vi "Main.vi"() -> ()   [LabVIEW 2024]
doc: "Main vi to run the Test Executive."
uses:
  <vilib>/Utility/miscctls.llb/LVRowAndColumnTypeDef.ctl
  <vilib>/addons/_JKI Toolkits/State Machine/_JKI_lib_State_Machine.llb/Select State(s)_err__jki_lib_state_machine.vi
  <vilib>/addons/_JKI Toolkits/State Machine/_JKI_lib_State_Machine.llb/Select State(s)_bool__jki_lib_state_machine.vi
  <vilib>/addons/_JKI Toolkits/State Machine/_JKI_lib_State_Machine.llb/Periodic Trigger__ogtk__JKI-SM__jki_lib_state_machine.vi
  <vilib>/Utility/file.llb/Read Delimited Spreadsheet (string).vi
  <userlib>/_OpenG.lib/file/file.llb/Strip Path Extension - String__ogtk.vi
  <userlib>/_OpenG.lib/lvzip/fileutil.llb/subVIs/FILE Rename (Path)__ogtk.vi
  <vilib>/Utility/file.llb/Write Delimited Spreadsheet (string).vi
  <vilib>/regexp/Match Regular Expression.xnode
  <userlib>/_OpenG.lib/appcontrol/appcontrol.llb/openg_application_control.lvlib
  <userlib>/_OpenG.lib/file/file.llb/openg_file.lvlib
  <userlib>/_OpenG.lib/string/string.llb/openg_string.lvlib
panel:
  in  "Abort Sequence":bool
  in  "Results":bool
  in  "TS Panel":bool
  in  "Tab Control":enum32{"TS", "R"}(tab)
  in  "SOF":bool caption="Checkbox"
  out "PassFail":string
  out "Sequence Name":string
  out "Status":string
  in  "Load Sequence":bool
  in  "Run Sequence":bool
  out "Sequence":string
  out "Operator":string
  out "Serial Number":string
  out "Results Table":string[][](table)
  in  "Exit":bool
  # "TEST EXECUTIVE V1"
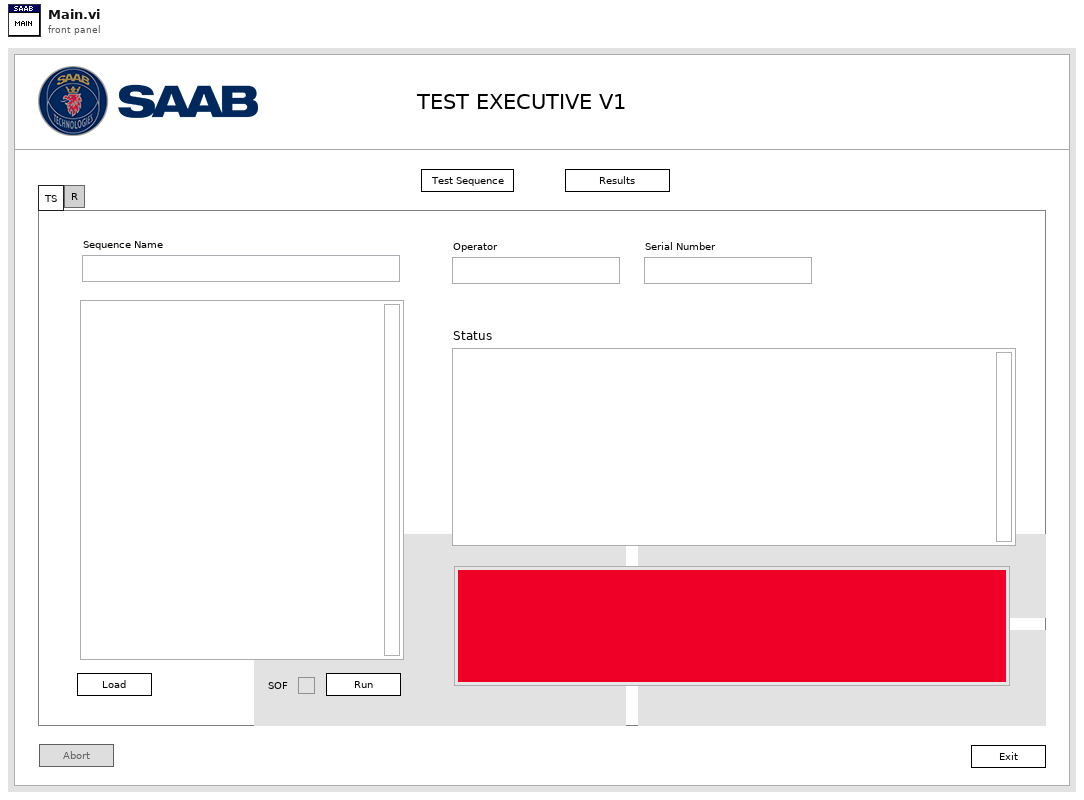
[diagram p1: front panel]
types:
  T1 = enum32{"Invalid", "Standard", "Closed", "Hidden", "Minimized", "Maximized"}
  T2 = enum32{"invalid app kind", "Development System", "Run Time System", "Student Edition", "Embedded LabVIEW", "Evaluation", "Custom"}
  T3 = cluster{"Core":cluster{"Current VI Reference":refnum<vi>, "Close Panel on Exit?":bool}, "Fail":bool, "Sequence Array":string[], "File Paths":cluster{"Seq File Path":path, "Limits File Path":path, "Results File Path":path, "Test File Path Array":path[]}, "Sequence Name":string, "Operator":string, "Serial Number":string, "Test Index":i32, "Test Time":dbl, "Start Seq TimeStamp ":cluster{"Start Seq Time":string, "Start Seq Date":string}, "End Seq Time":string, "Status":string, "SOF":bool, "Abort":bool, "Reference Array":refnum<vi>[]}
  T4 = cluster{"Start Seq Time":string, "Start Seq Date":string}
  T5 = cluster{"Seq File Path":path, "Limits File Path":path, "Results File Path":path, "Test File Path Array":path[]}
  T6 = cluster{"Current VI Reference":refnum<vi>, "Close Panel on Exit?":bool}
  T7 = enum8{"Enabled", "Disabled", "Disabled and Grayed Out"}
  T8 = typedef "LVRowAndColumnTypeDef.ctl" = cluster{"Row":i32, "Column":i32}
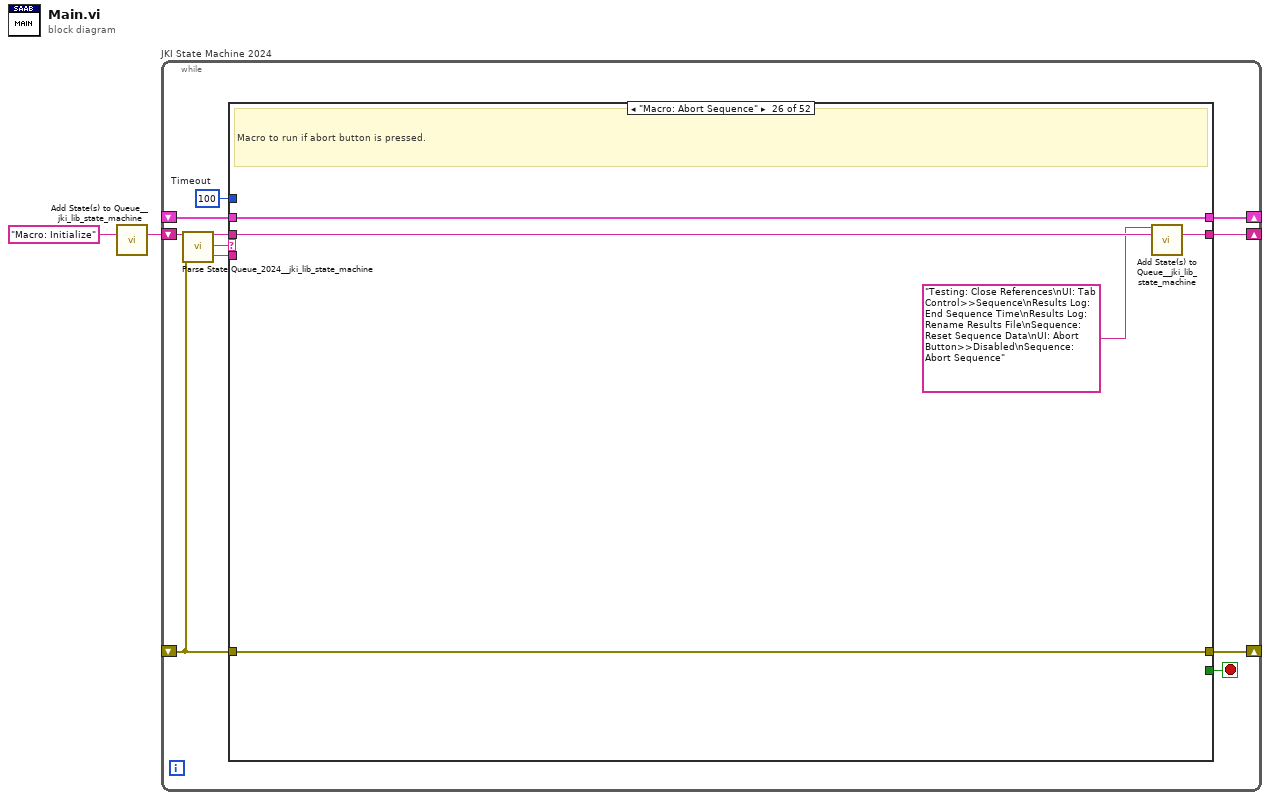
[diagram p0: block diagram]
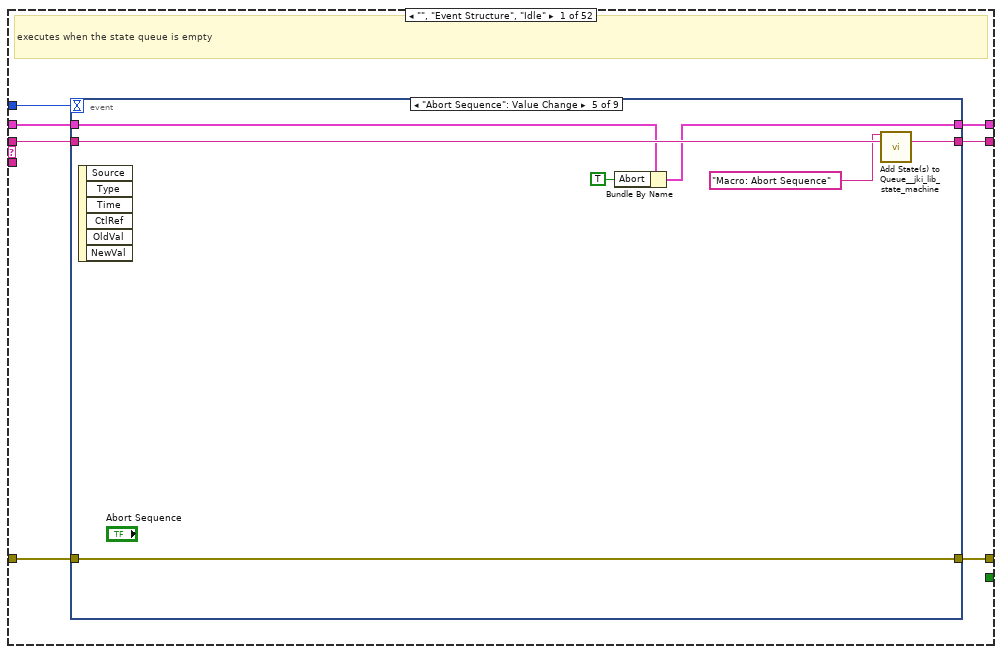
[diagram p2: hidden frame]
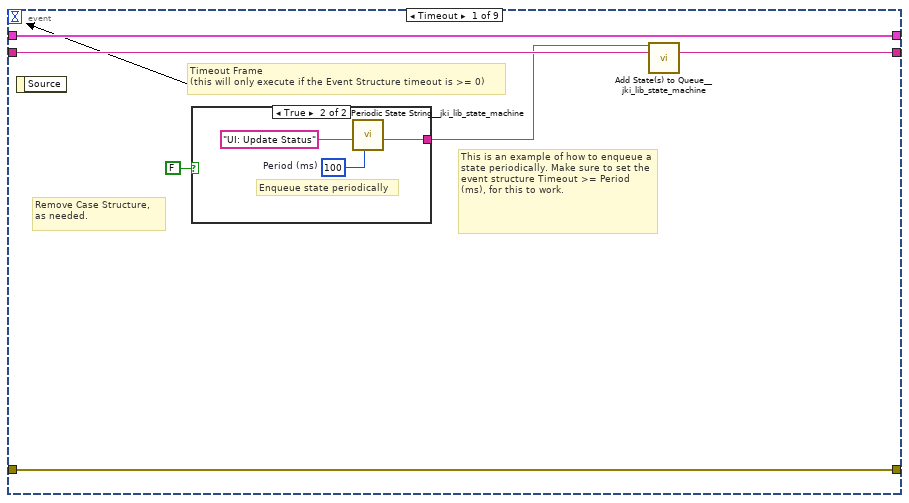
[diagram p3: hidden frame]
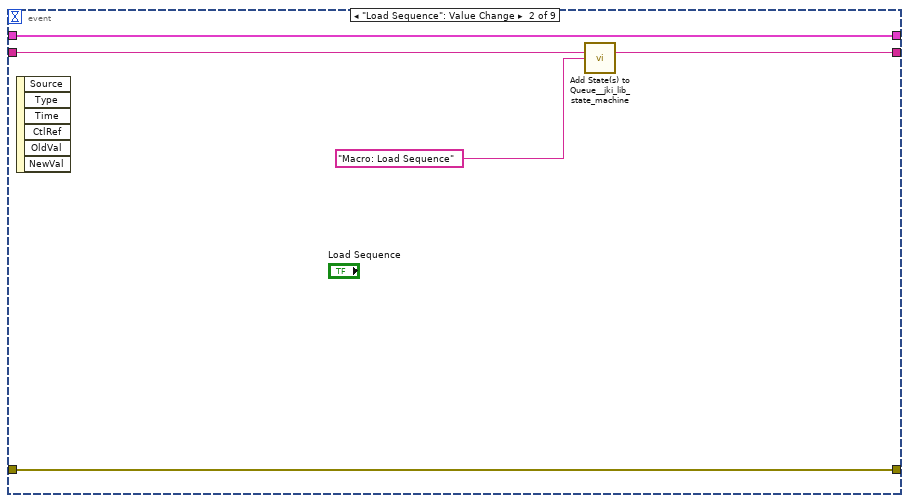
[diagram p5: hidden frame]
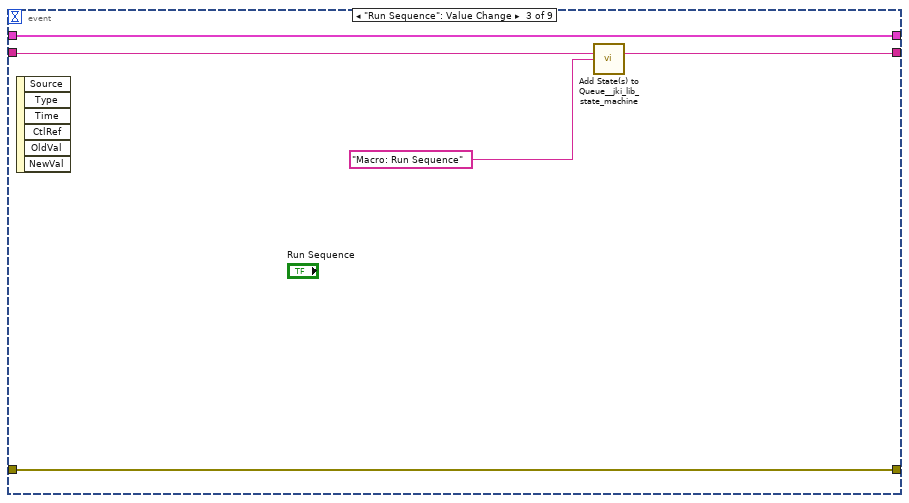
[diagram p6: hidden frame]
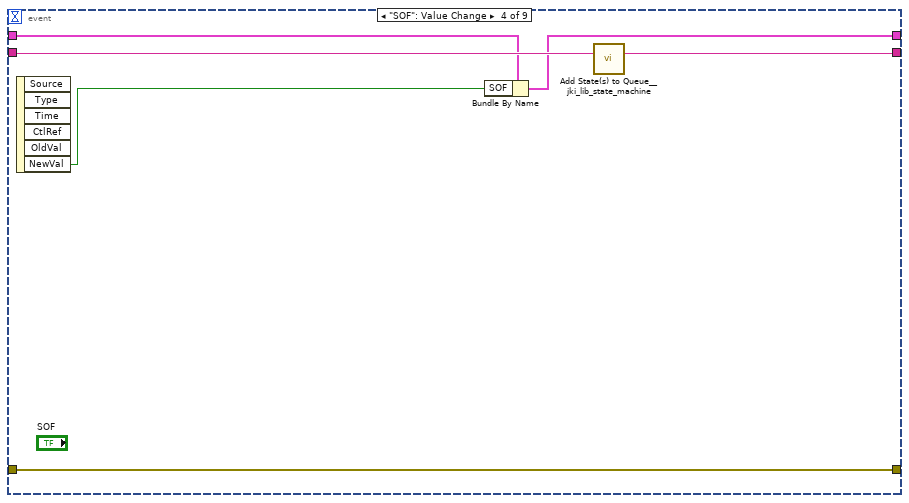
[diagram p7: hidden frame]
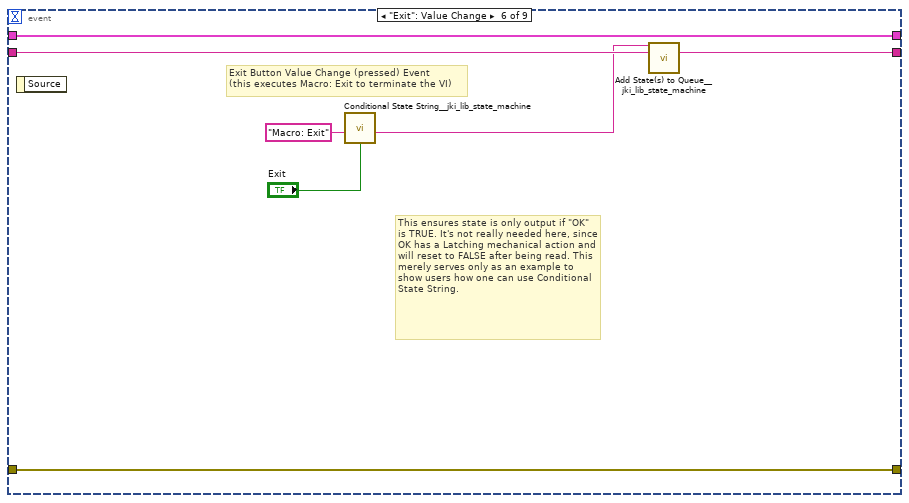
[diagram p8: hidden frame]
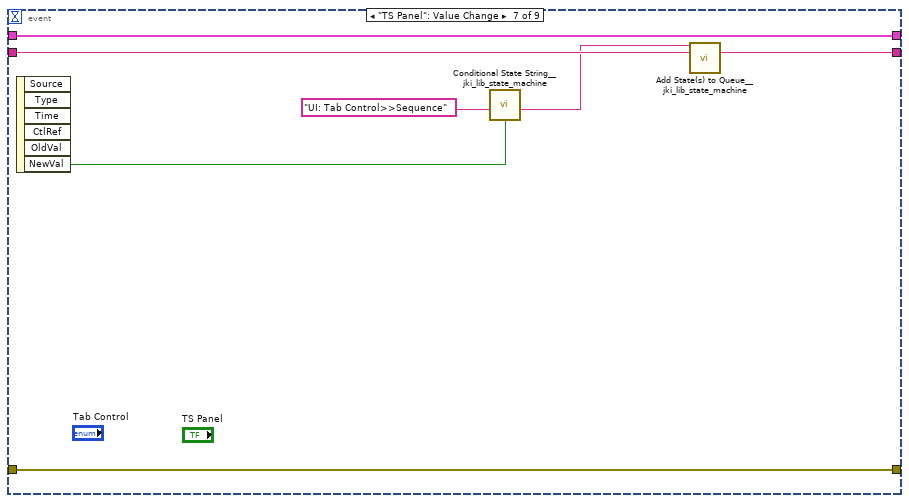
[diagram p9: hidden frame]
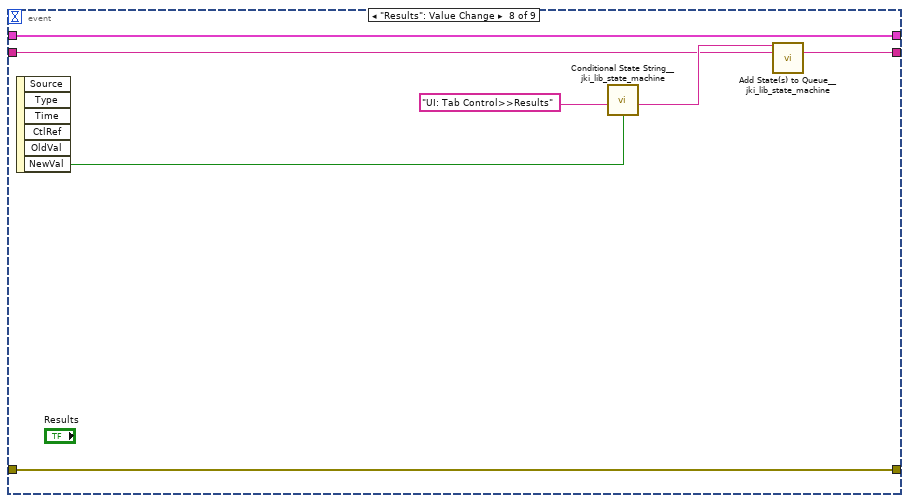
[diagram p10: hidden frame]
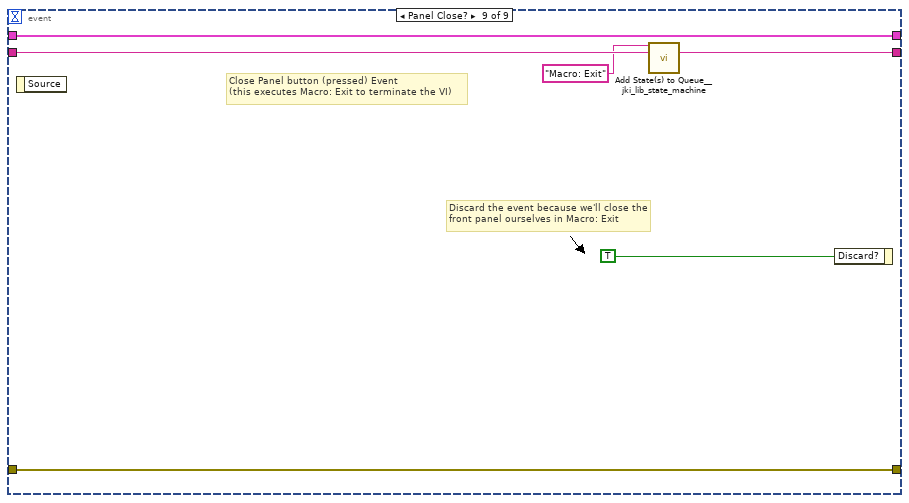
[diagram p11: hidden frame]
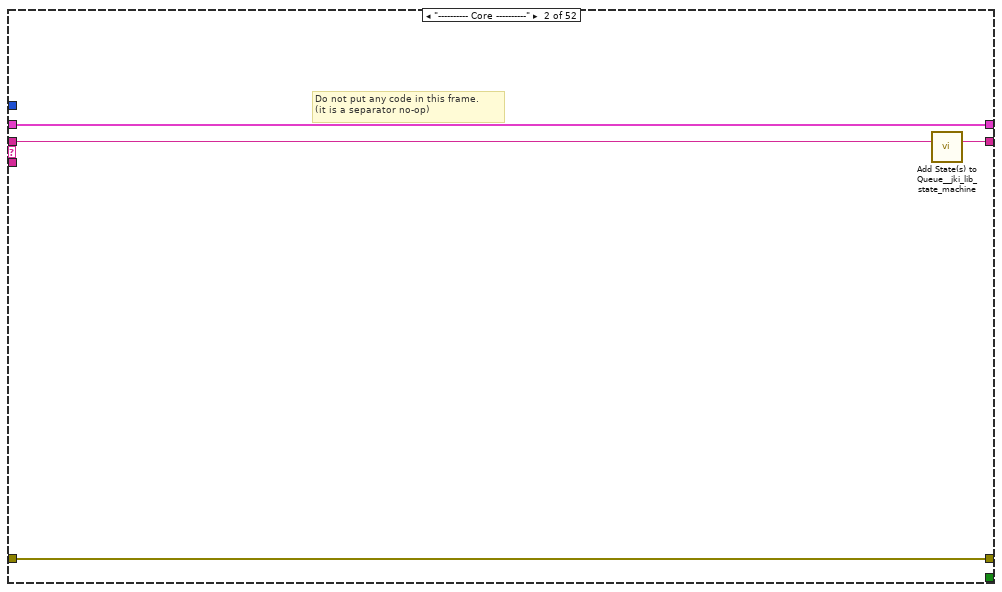
[diagram p12: hidden frame]
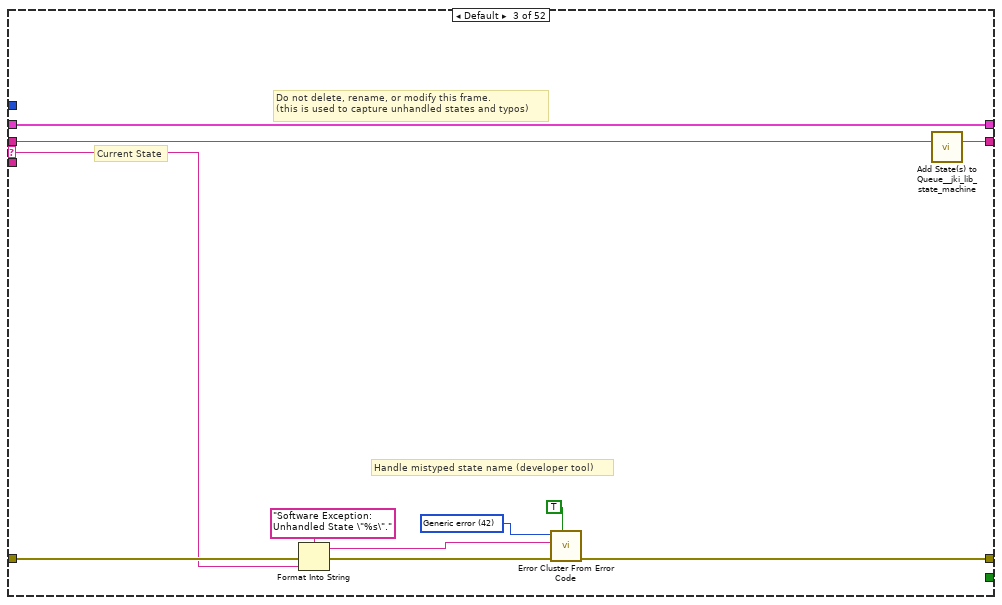
[diagram p13: hidden frame]
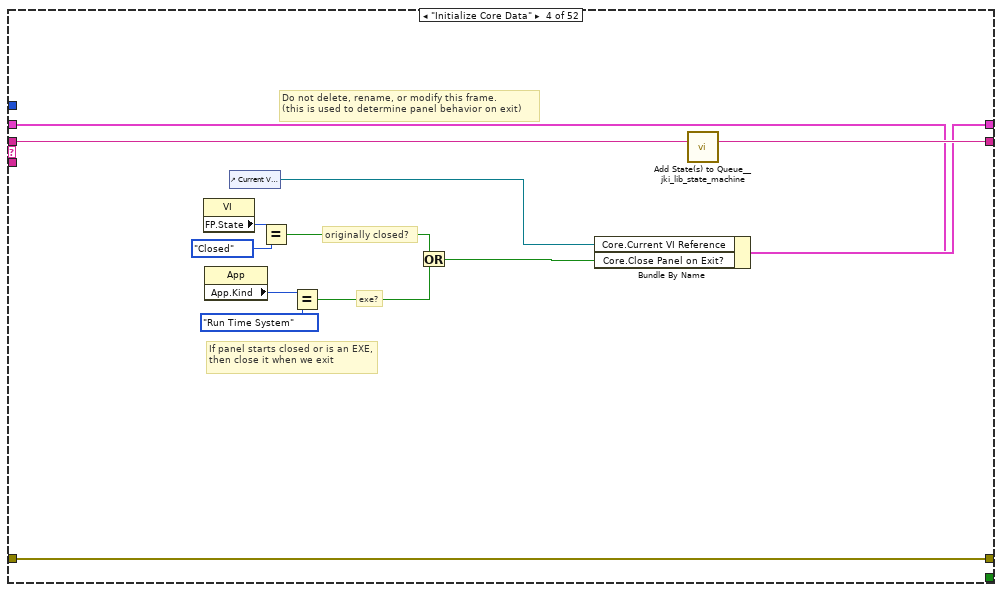
[diagram p14: hidden frame]
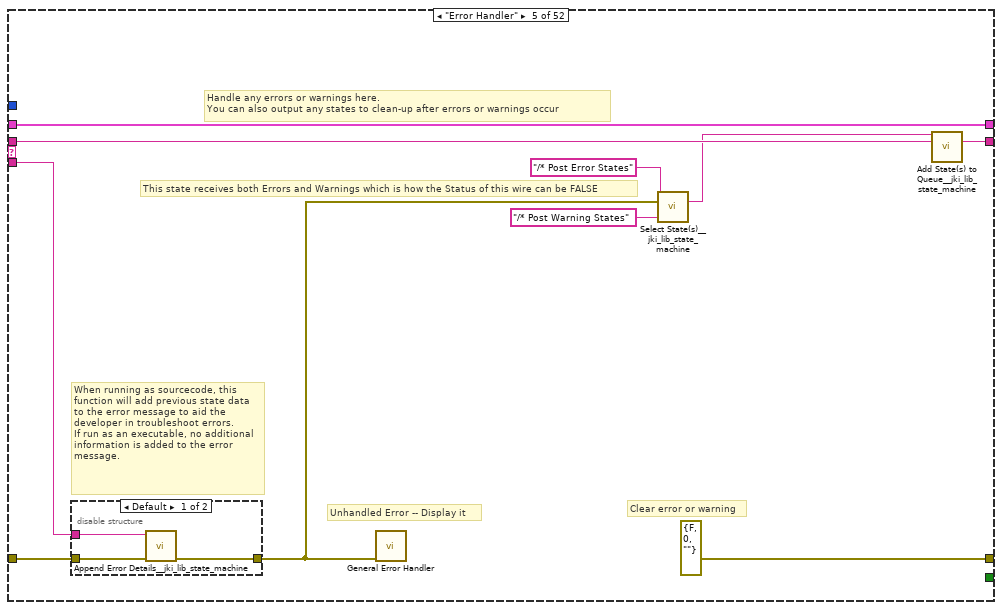
[diagram p15: hidden frame]
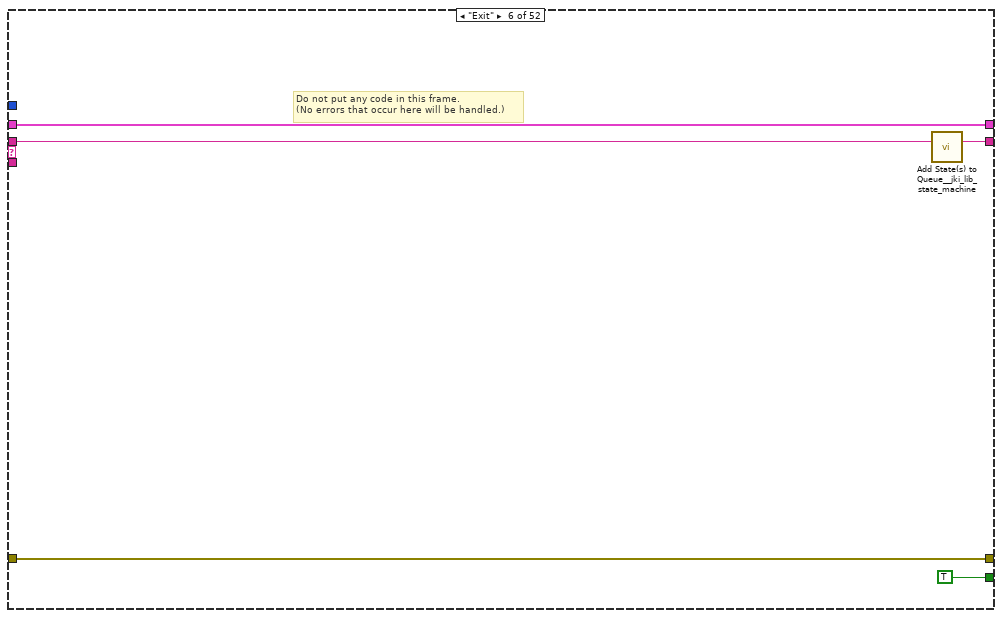
[diagram p17: hidden frame]
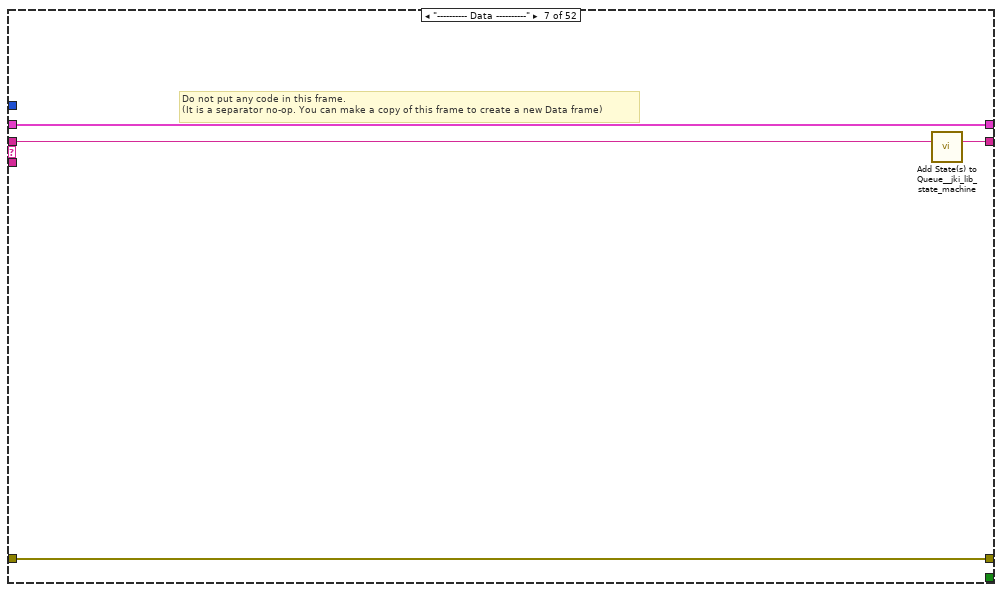
[diagram p18: hidden frame]
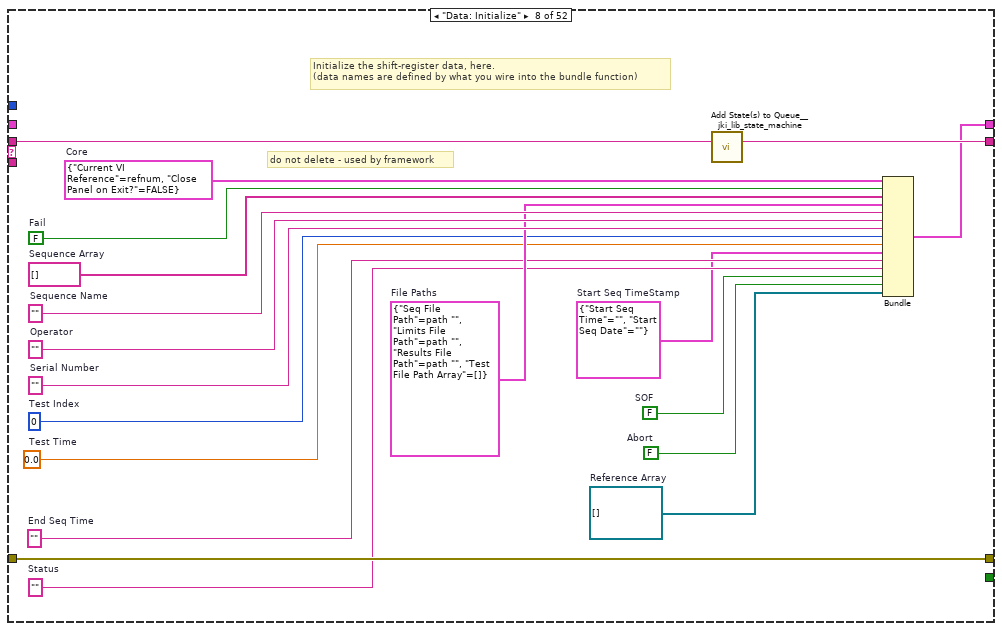
[diagram p19: hidden frame]
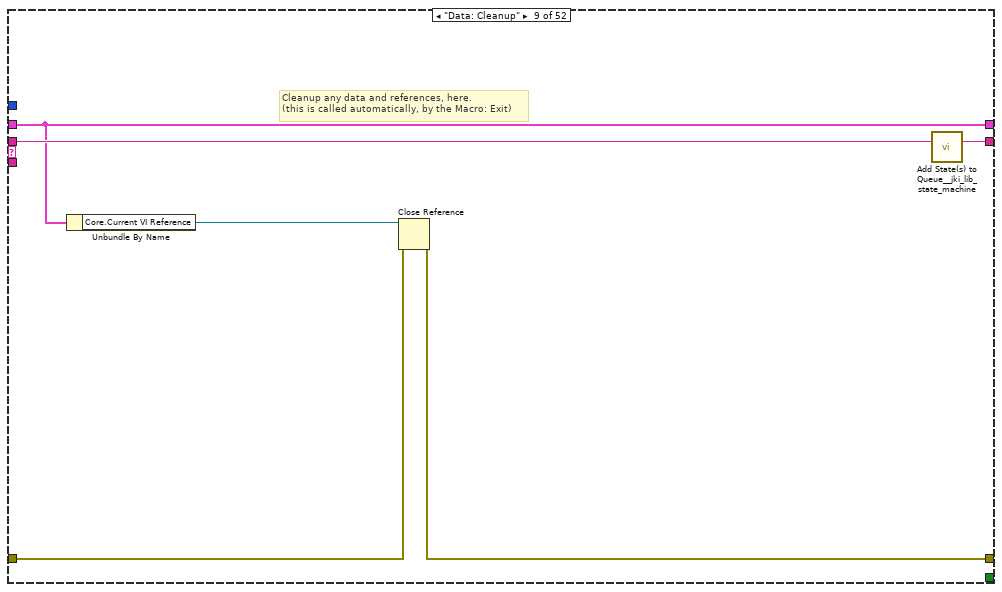
[diagram p20: hidden frame]
diagram:
  n1 = call <vilib>:"Add State(s) to Queue__jki_lib_state_machine.vi"("State(s) in (\"\")"="Macro: Initialize") -> ("States Out"=w2:string)  [unwired: 14 in]
  n2 = while "JKI State Machine 2024" {
    shift-right: [w6] -> _
    shift-left: _ -> [w5]
    shift-right: [w9] -> _
    shift-left: _ -> [w3]
    shift-right: [w8] -> _
    shift-left: w2 -> [w10]
    stop <- w7 stop-if-true
    w4 = 100  # Timeout
    n3 = call <vilib>:"Parse State Queue_2024__jki_lib_state_machine.vi"("State Queue"=w10, "Error In (no error)"=w3) -> ("Remaining States"=w12:string, "Current State"=w13:string, "Arguments"=w11:string)  [unwired: 11 in]
    n4 = case shown="\"Macro: Abort Sequence\"" w13 {
      selector: w13 -> [_ _ w84 _ _ _ _ _ _ _ _ _ _ _ _ _ _ _ _ _ _ _ _ _ _ _ _ _ _ _ _ _ _ _ _ _ _ _ _ _ _ _ _ _ _ _ _ _ _ _ _ _]
      tunnel: w12 -> [w20 w83 w88 w107 w117 w126 w130 w149 w155 w159 w169 w177 w195 w209 w220 w232 w241 w252 w258 w269 w338 w343 w348 w353 w358 w363 w368 w377 w381 w398 w413 w424 _ w431 w454 w462 w474 w492 w513 w522 w539 w580 w714 w731 w737 w755 w768 w783 w790 w799 w817 w825]
      tunnel: w11 -> [_ _ _ _ w112 _ _ _ _ _ _ w170 _ _ w215 _ _ w243 w253 w263 _ _ _ _ _ _ _ _ _ _ _ _ _ _ _ _ _ _ _ _ _ _ _ _ _ _ _ _ _ _ _ _]
      tunnel: w5 -> [w18 w80 w86 w100 w114 w124 w127 _ w150 w156 w167 w175 w192 w207 w218 w230 w239 w250 w256 w265 w335 w340 w345 w350 w354 w359 w365 w375 w378 w391 w408 w422 w425 w437 w452 w460 w471 w487 w511 w518 w528 w578 w710 w728 w744 w752 w765 w776 w786 w793 w807 w823]
      tunnel: [w17 w81 w90 w104 errorcluster {"status"=FALSE, "code"=0, "source"=""} ("error out") w123 w128 w144 w151 w157 w164 w174 w182 w205 w217 w223 w235 w249 w254 w266 w336 w341 w346 w351 w356 w361 w366 w372 w379 w385 w411 w420 w426 w433 w450 w455 w472 w489 w499 w520 w531 w562 w712 w722 w738 w753 w766 w781 w788 w797 w813 w820] -> w9
      tunnel: w3 -> [w14 w81 w89 w104 w113 w123 w128 w144 w152 w157 w162 w172 w193 w206 w216 w229 w238 w248 w255 w267 w336 w341 w346 w351 w356 w361 w366 w372 w379 w392 w411 w420 w429 w433 w450 w458 w472 w489 w510 w520 w534 w571 w712 w727 w742 w753 w766 w781 w788 w797 w812 w819]
      tunnel: [w19 w82 w87 w106 w116 w125 w129 w148 w154 w158 w168 w176 w194 w208 w219 w231 w240 w251 w257 w268 w337 w342 w347 w352 w357 w362 w367 w376 w380 w397 w412 w423 w430 w438 w453 w461 w473 w491 w512 w521 w538 w579 w713 w730 w745 w754 w767 w782 w789 w798 w816 w824] -> w8
      tunnel: [_ _ _ _ _ TRUE _ _ _ _ _ _ _ _ _ _ _ _ _ _ _ _ _ _ _ _ _ _ _ _ _ _ _ _ _ _ _ _ _ _ _ _ _ _ _ _ _ _ _ _ _ _] -> w7
      tunnel: [w16 w80 w86 w105 w114 w124 w127 w147 w150 w156 w167 w175 w192 w207 w218 w230 w239 w250 w256 w265 w335 w340 w345 w350 w354 w359 w365 w375 w378 w390 w408 w421 w425 w436 w451 w459 w471 w490 w511 w517 w527 w578 w709 w729 w743 w752 w765 w775 w785 w792 w806 w822] -> w6
      tunnel: w4 -> [w15 _ _ _ _ _ _ _ _ _ _ _ _ _ _ _ _ _ _ _ _ _ _ _ _ _ _ _ _ _ _ _ _ _ _ _ _ _ _ _ _ _ _ _ _ _ _ _ _ _ _ _]
      frame "", "Event Structure", "Idle" {
        # "executes when the state queue is empty"
        n5 = event shown="[4] \"Abort Sequence\": Value Change" {
          selector: _ -> [_ _ _ _ _ _ _ _ _]
          dyn-events: _ -> [_ _ _ _ _ _ _ _ _]
          timeout: w15 -> [_ _ _ _ _ _ _ _ _]
          tunnel: w20 -> [w26 w30 w37 w44 w50 w59 w64 w69 w79]
          tunnel: [w25 w33 w38 w45 w51 w58 w65 w71 w78] -> w19
          tunnel: w18 -> [w23 w31 w36 w41 w48 w56 w66 w73 w76]
          tunnel: [w24 w34 w35 w43 w52 w57 w60 w67 w77] -> w17
          tunnel: w14 -> [w24 w34 w35 w43 w52 w57 w60 w67 w77]
          tunnel: [w23 w31 w36 w42 w47 w56 w66 w73 w76] -> w16
          event Timeout {
            # "Remove Case Structure, as needed."
            # "This is an example of how to enqueue a state periodically. Make sure to set the event structure Timeout >= Period (ms), for this to work."
            # "Timeout Frame\n(this will only execute if the Event Structure timeout is >= 0)"
            n6 = event-data() -> ()  [unwired: 1 in, 1 out]
            n7 = case shown="True" FALSE {
              tunnel: [_ w29] -> w22
              frame False {
              }
              frame True {
                w27 = u32 100  # Period (ms)
                # "Enqueue state periodically"
                n8 = call <vilib>:"Periodic State String__jki_lib_state_machine.vi"("Period (ms)"=w27, "State"="UI: Update Status") -> ("State Out"=w29:string)  [unwired: 9 in]
              }
            }
            n9 = call <vilib>:"Add State(s) to Queue__jki_lib_state_machine.vi"("State(s) in Front (\"\")"=w22, "State(s) in (\"\")"=w26) -> ("States Out"=w25:string)  [unwired: 13 in]
          }
          event "Load Sequence": Value Change {
            n10 = event-data() -> ()  [unwired: 1 in, 6 out]
            n11 = call <vilib>:"Add State(s) to Queue__jki_lib_state_machine.vi"("State(s) in (\"\")"=w30, "State(s) at Back (\"\")"="Macro: Load Sequence" ("State(s) at Back (\"\")")) -> ("States Out"=w33:string)  [unwired: 13 in]
          }
          event "Run Sequence": Value Change {
            n12 = event-data() -> ()  [unwired: 1 in, 6 out]
            n13 = call <vilib>:"Add State(s) to Queue__jki_lib_state_machine.vi"("State(s) in (\"\")"=w37, "State(s) at Back (\"\")"="Macro: Run Sequence" ("State(s) at Back (\"\")")) -> ("States Out"=w38:string)  [unwired: 13 in]
          }
          event "SOF": Value Change {
            n14 = event-data() -> ("NewVal"=w40:bool)  [unwired: 1 in, 5 out]
            n15 = Bundle By Name(cluster=w41, "SOF"=w40) -> (w42:T3)
            n16 = call <vilib>:"Add State(s) to Queue__jki_lib_state_machine.vi"("State(s) in (\"\")"=w44) -> ("States Out"=w45:string)  [unwired: 14 in]
          }
          event "Abort Sequence": Value Change {
            n17 = event-data() -> ()  [unwired: 1 in, 6 out]
            n18 = Bundle By Name(cluster=w48, "Abort"=TRUE) -> (w47:T3)
            n19 = call <vilib>:"Add State(s) to Queue__jki_lib_state_machine.vi"("State(s) in Front (\"\")"="Macro: Abort Sequence", "State(s) in (\"\")"=w50) -> ("States Out"=w51:string)  [unwired: 13 in]
          }
          event "Exit": Value Change {
            # "This ensures state is only output if \"OK\" is TRUE. It's not really needed here, since OK has a Latching mechanical action and will reset to FALSE after being read. This merely serves only as an example to show users how one can use Conditional State String."
            # "Exit Button Value Change (pressed) Event\n(this executes Macro: Exit to terminate the VI)"
            n20 = event-data() -> ()  [unwired: 1 in, 1 out]
            n21 = call <vilib>:"Conditional State String__jki_lib_state_machine.vi"("Do State(s)?"="Exit", "State"="Macro: Exit") -> ("State Out"=w53:string)  [unwired: 7 in]
            n22 = call <vilib>:"Add State(s) to Queue__jki_lib_state_machine.vi"("State(s) in Front (\"\")"=w53, "State(s) in (\"\")"=w59) -> ("States Out"=w58:string)  [unwired: 13 in]
          }
          event "TS Panel": Value Change {
            n23 = event-data() -> ("NewVal"=w62:bool)  [unwired: 1 in, 5 out]
            n24 = call <vilib>:"Conditional State String__jki_lib_state_machine.vi"("Do State(s)?"=w62, "State"="UI: Tab Control>>Sequence") -> ("State Out"=w63:string)  [unwired: 7 in]
            n25 = call <vilib>:"Add State(s) to Queue__jki_lib_state_machine.vi"("State(s) in Front (\"\")"=w63, "State(s) in (\"\")"=w64) -> ("States Out"=w65:string)  [unwired: 13 in]
          }
          event "Results": Value Change {
            n26 = event-data() -> ("NewVal"=w68:bool)  [unwired: 1 in, 5 out]
            n27 = call <vilib>:"Conditional State String__jki_lib_state_machine.vi"("Do State(s)?"=w68, "State"="UI: Tab Control>>Results") -> ("State Out"=w70:string)  [unwired: 7 in]
            n28 = call <vilib>:"Add State(s) to Queue__jki_lib_state_machine.vi"("State(s) in Front (\"\")"=w70, "State(s) in (\"\")"=w69) -> ("States Out"=w71:string)  [unwired: 13 in]
          }
          event Panel Close? {
            # "Discard the event because we'll close the front panel ourselves in Macro: Exit"
            # "Close Panel button (pressed) Event\n(this executes Macro: Exit to terminate the VI)"
            n29 = event-data() -> ()  [unwired: 1 in, 1 out]
            n30 = call <vilib>:"Add State(s) to Queue__jki_lib_state_machine.vi"("State(s) in Front (\"\")"="Macro: Exit", "State(s) in (\"\")"=w79) -> ("States Out"=w78:string)  [unwired: 13 in]
            n31 = event-data("Discard?"=TRUE) -> ()  [unwired: 1 in, 1 out]
          }
        }
      }
      frame "---------- Core ----------" {
        # "Do not put any code in this frame.\n(it is a separator no-op)"
        n32 = call <vilib>:"Add State(s) to Queue__jki_lib_state_machine.vi"("State(s) in (\"\")"=w83) -> ("States Out"=w82:string)  [unwired: 14 in]
      }
      frame Default {
        w93 = 42 items=["No error", "Argument error", "Memory is full", "Out of zone", "End of file", "File already open", "Generic file I/O error", "File not found", "File permission error", "Disk is full", "Duplicate path", "Too many files open", "System feature not enabled", "Resource file not found", "Cannot add resource", "Resource not found", "Image not found", "Image memory error", "Pen does not exist", "Config type invalid", "Config token not found", "Config parse error", "Config memory error", "Bad external code format", "Bad external code offset", "External code not present", "Null window", "Destroy window error", "Null menu", "Print aborted", "Bad print record", "Print driver error", "Windows error during printing", "Memory error during printing", "Print dialog error", "Generic print error", "Invalid device refnum", "Device not found", "Device parameter error", "Device unit error", "Cannot open device", "Device call aborted", "Generic error", "Cancelled by user", "Object ID too low", "Object ID too high", "Object not in heap", "Unknown heap", "Unknown object (invalid DefProc)", "Unknown object (DefProc not in table)", "Message out of range", "Invalid (null) method", "Unknown message", "Manager call not supported", "Bad address", "Network operation in progress", "Network operation timed out", "Connection is busy", "Network attribute not supported", "Network error", "Address in use", "System out of memory", "Connection aborted", "Connection refused", "Not connected", "Already connected", "Connection closed", "Initialization error (interapplication manager)", "Bad occurrence", "Wait on unbound occurrence handler", "Occurrence queue overflow", "Datalog type conflict", "Unused", "Unrecognized type (interapplication manager)", "Memory corrupt", "Failed to make temporary DLL", "Old CIN version", "Drag socket not found", "Failed to load drop-object", "Failed to register OLE object", "Failed to release OLE object", "Format specifier type mismatch", "Unknown format specifier", "Too few format specifiers", "Too many format specifiers", "Scan failed", "Newer CIN version", "Error converting to variant", "Runtime menu error", "Password tampered", "Variant attribute not found", "Incompatible variant data type", "Event data is not available", "Event Store is not present", "Occurrence is not found", "Event Queue is not created", "Event info is not available", "Refnum passed is NULL", "Error retrieving Class GUID", "Error retrieving CoClass GUID", "Error retrieving TypeLib GUID.", "Bad built application magic bytes.", "Specific driver is different from the specific driver associated with the Logical Name.", "There is no session opened to the class driver.", "Max Error", "MAX - Error with config objects", "MAX - Error loading configuration", "MAX - Group not supported"]
        # "Current State"
        # "Do not delete, rename, or modify this frame.\n(this is used to capture unhandled states and typos)"
        # "Handle mistyped state name (developer tool)"
        n33 = Format Into String(format string="Software Exception: Unhandled State \"%s\"." ("message"), error in=w89, w84) -> (resulting string=w92:string, error out=w91:errorcluster)  [unwired: 1 in]
        n34 = call <vilib>:"Error Cluster From Error Code.vi"("show call chain? (False)"=TRUE, "error in (no error)"=w91, "error message (\"\")"=w92, "error code (0)"=w93) -> ("error out"=w90:errorcluster)  [unwired: 5 in]
        n35 = call <vilib>:"Add State(s) to Queue__jki_lib_state_machine.vi"("State(s) in (\"\")"=w88) -> ("States Out"=w87:string)  [unwired: 14 in]
      }
      frame "Initialize Core Data" {
        # "Do not delete, rename, or modify this frame.\n(this is used to determine panel behavior on exit)"
        # "originally closed?"
        # "exe?"
        # "If panel starts closed or is an EXE, then close it when we exit"
        n36 = property class="VI"() -> ("FP.State"=w97:T1)  [unwired: 2 in, 2 out]
        n37 = property class="App"() -> ("App.Kind"=w103:T2)  [unwired: 2 in, 2 out]
        n38 = control-ref of="Current VI Reference"() -> (w98:refnum<vi>)
        n39 = Equal?(x=w97, y=T1."Closed" ("Front Panel Window:State")) -> (x = y?=w95:bool)
        n40 = Equal?(x=w103, y=T2."Run Time System" ("Application:Kind")) -> (x = y?=w101:bool)
        n41 = Or(x=w95, y=w101) -> (x .or. y?=w99:bool)
        n42 = Bundle By Name(cluster=w100, "Core.Current VI Reference"=w98, "Core.Close Panel on Exit?"=w99) -> (w105:T3)
        n43 = call <vilib>:"Add State(s) to Queue__jki_lib_state_machine.vi"("State(s) in (\"\")"=w107) -> ("States Out"=w106:string)  [unwired: 14 in]
      }
      frame "Error Handler" {
        # "When running as sourcecode, this function will add previous state data to the error message to aid the developer in troubleshoot errors.\nIf run as an executable, no additional information is added to the error message."
        # "This state receives both Errors and Warnings which is how the Status of this wire can be FALSE"
        # "Unhandled Error -- Display it"
        # "Handle any errors or warnings here.\nYou can also output any states to clean-up after errors or warnings occur"
        # "Clear error or warning"
        n44 = disable-structure shown="Default" {
          disable-tunnel: w113 -> [w120 w121]
          disable-tunnel: w112 -> [w119 _]
          disable-tunnel: [w118 w121] -> w111
          frame condition #0 (active) {
            n45 = call <vilib>:"Append Error Details__jki_lib_state_machine.vi"("error in (no error)"=w120, "Previous State and Argument(s)"=w119) -> ("error out"=w118:errorcluster)  [unwired: 9 in]
          }
          frame condition #1 {
          }
        }
        n46 = call <vilib>:"General Error Handler.vi"("error in (no error)"=w111) -> ()  [unwired: 10 in, 5 out]
        n47 = call-poly <vilib>:"Select State(s)__jki_lib_state_machine.vi"("State(s) if True (\"\")"="/* Post Error States", "Select"=w111, "State(s) if False (\"\")"="/* Post Warning States") -> ("States Out"=w109:string)  [unwired: 12 in]
        n48 = call <vilib>:"Add State(s) to Queue__jki_lib_state_machine.vi"("State(s) in Front (\"\")"=w109, "State(s) in (\"\")"=w117) -> ("States Out"=w116:string)  [unwired: 13 in]
      }
      frame "Exit" {
        # "Do not put any code in this frame.\n(No errors that occur here will be handled.)"
        n49 = call <vilib>:"Add State(s) to Queue__jki_lib_state_machine.vi"("State(s) in (\"\")"=w126) -> ("States Out"=w125:string)  [unwired: 14 in]
      }
      frame "---------- Data ----------" {
        # "Do not put any code in this frame.\n(It is a separator no-op. You can make a copy of this frame to create a new Data frame)"
        n50 = call <vilib>:"Add State(s) to Queue__jki_lib_state_machine.vi"("State(s) in (\"\")"=w130) -> ("States Out"=w129:string)  [unwired: 14 in]
      }
      frame "Data: Initialize" {
        w131 = refnum<vi>[] []  # Reference Array
        w132 = FALSE  # Abort
        w133 = FALSE  # SOF
        w134 = T4 {"Start Seq Time"="", "Start Seq Date"=""}  # Start Seq TimeStamp
        w135 = ""  # Status
        w136 = ""  # End Seq Time
        w137 = 0.0  # Test Time
        w138 = 0  # Test Index
        w139 = T5 {"Seq File Path"=path "", "Limits File Path"=path "", "Results File Path"=path "", "Test File Path Array"=[]}  # File Paths
        w140 = string[] []  # Sequence Array
        w141 = ""  # Serial Number
        w142 = ""  # Operator
        w143 = ""  # Sequence Name
        w145 = T6 {"Current VI Reference"=refnum, "Close Panel on Exit?"=FALSE}  # Core
        w146 = FALSE  # Fail
        # "do not delete - used by framework"
        # "Initialize the shift-register data, here.\n(data names are defined by what you wire into the bundle function)"
        n51 = call <vilib>:"Add State(s) to Queue__jki_lib_state_machine.vi"("State(s) in (\"\")"=w149) -> ("States Out"=w148:string)  [unwired: 14 in]
        n52 = Bundle("Core"=w145, "Fail"=w146, "Sequence Array"=w140, "File Paths"=w139, "Sequence Name"=w143, "Operator"=w142, "Serial Number"=w141, "Test Index"=w138, "Test Time"=w137, "Start Seq TimeStamp"=w134, "End Seq Time"=w136, "Status"=w135, "SOF"=w133, "Abort"=w132, "Reference Array"=w131) -> (w147:T3)  [unwired: 1 in]
      }
      frame "Data: Cleanup" {
        # "Cleanup any data and references, here.\n(this is called automatically, by the Macro: Exit)"
        n53 = Unbundle By Name(w150) -> ("Core.Current VI Reference"=w153:refnum<vi>)
        n54 = Close Reference(reference=w153, error in (no error)=w152) -> (error out=w151:errorcluster)
        n55 = call <vilib>:"Add State(s) to Queue__jki_lib_state_machine.vi"("State(s) in (\"\")"=w155) -> ("States Out"=w154:string)  [unwired: 14 in]
      }
      frame "---------- UI ----------" {
        # "Do not put any code in this frame.\n(It is a separator no-op. You can make a copy of this frame to create a new UI frame)"
        n56 = call <vilib>:"Add State(s) to Queue__jki_lib_state_machine.vi"("State(s) in (\"\")"=w159) -> ("States Out"=w158:string)  [unwired: 14 in]
      }
      frame "UI: Initialize" {
        w160 = FALSE  # SOF
        w163 = enum32{"TS", "R"}."TS"  # Tab Control
        # "Initialize the User Interface, here.\n(this is called automatically, by the Macro: Initialize)"
        n57 = property on="SOF" class="Bool (strict)"(error in=w162, "Value"=w160) -> (error out=w161:errorcluster)  [unwired: 1 in, 1 out]
        n58 = property on="Tab Control" class="TabCtl (strict)"(error in=w161, "Tabs Visible?"=FALSE, "Value"=w163) -> (error out=w165:errorcluster)  [unwired: 1 in, 1 out]
        n59 = call <userlib>:"Fit VI window to Largest Dec__ogtk.vi"("error in (no error)"=w165) -> ("error out"=w164:errorcluster)  [unwired: 5 in, 1 out]
        n60 = call <vilib>:"Add State(s) to Queue__jki_lib_state_machine.vi"("State(s) in (\"\")"=w169) -> ("States Out"=w168:string)  [unwired: 14 in]
      }
      frame "UI: Tab Control" {
        # "Selects the tab defined by the state argument"
        n61 = case shown="\"Sequence\", Default" w170 {
          tunnel: [w179 w181] -> w173
          tunnel: w172 -> [w178 w180]
          tunnel: [w178 w180] -> w171
          frame "Results" {
            w179 = enum32{"TS", "R"}."R"  # Tab Control
          }
          frame "Sequence", Default {
            w181 = enum32{"TS", "R"}."TS"  # Tab Control
          }
        }
        n62 = property on="Tab Control" class="TabCtl (strict)"(error in=w171, "Value"=w173) -> (error out=w174:errorcluster)  [unwired: 1 in, 1 out]
        n63 = call <vilib>:"Add State(s) to Queue__jki_lib_state_machine.vi"("State(s) in (\"\")"=w177) -> ("States Out"=w176:string)  [unwired: 14 in]
      }
      frame "UI: Update Status" {
        # "Update the status on the FP. Build the text for the status string and add any failures. Display a big passfail string box and colour appropriatly."
        n64 = Unbundle By Name(w192) -> ("Start Seq TimeStamp.Start Seq Date"=w190:string, "Start Seq TimeStamp.Start Seq Time"=w189:string, "End Seq Time"=w188:string, "File Paths.Results File Path"=w191:path)
        n65 = call "Search for Fail.vi"("Results File Path"=w191, "error in (no error)"=w193) -> ("String"=w186:string, "Pass Status"=w184:bool, "error out"=w185:errorcluster)  [unwired: 11 in]
        n66 = case shown="False" w184 {
          tunnel: w185 -> [w198 w202]
          tunnel: ["FAIL" "PASS"] -> w183
          tunnel: [w197 w201] -> w182
          frame False {
            n67 = property on="PassFail" class="Str"(error in=w198, "Text.BGColor"=u32 15663143) -> (error out=w197:errorcluster)  [unwired: 1 in, 1 out]
          }
          frame True {
            n68 = property on="PassFail" class="Str"(error in=w202, "Text.BGColor"=u32 51250) -> (error out=w201:errorcluster)  [unwired: 1 in, 1 out]
          }
        }
        "PassFail" <- w183
        n69 = call "Build Text2"("Fail"=w186, "Date"=w190, "Start"=w189, "Finish"=w188) -> ("Result"=→"Status":string)  [unwired: 10 in, 1 out]
        n70 = call <vilib>:"Add State(s) to Queue__jki_lib_state_machine.vi"("State(s) in (\"\")"=w195) -> ("States Out"=w194:string)  [unwired: 14 in]
      }
      frame "UI: Uninitialize" {
        # "Cleanup the User Interface, here.\n(this is called automatically, by the Macro: Exit)"
        n71 = property on="Tab Control" class="TabCtl (strict)"(error in=w206, "Tabs Visible?"=TRUE) -> (error out=w205:errorcluster)  [unwired: 1 in, 1 out]
        n72 = call <vilib>:"Add State(s) to Queue__jki_lib_state_machine.vi"("State(s) in (\"\")"=w209) -> ("States Out"=w208:string)  [unwired: 14 in]
      }
      frame "UI: Run Button" {
        w212 = T7."Disabled and Grayed Out"  # Disabled
        w213 = T7."Enabled"  # Disabled
        # "Enables or disabled the Run button based on state arguments."
        n73 = Equal?(x=w215, y="Disabled") -> (x = y?=w214:bool)
        n74 = Select(t=w212, s=w214, f=w213) -> (s? t:f=w210:T7)
        n75 = property on="Run Sequence" class="Bool"(error in=w216, "DisabledEnum"=w210) -> (error out=w217:errorcluster)  [unwired: 1 in, 1 out]
        n76 = call <vilib>:"Add State(s) to Queue__jki_lib_state_machine.vi"("State(s) in (\"\")"=w220) -> ("States Out"=w219:string)  [unwired: 14 in]
      }
      frame "UI: Init Results Table" {
        w222 = T8 {"Row"=-1, "Column"=-2}  # Active Cell:Active Cell
        w225 = string[] ["Test Name", "Sub Test", "Step Type", "Comparison Type", "Lower Limit", "Upper Limit", "Measurment", "Status"]  # Row Header Strings[]
        w226 = string[][] []  # Table
        w228 = T8 {"Row"=-2, "Column"=-2}  # Active Cell:Active Cell
        # "Initialise the results table on the FP to clear previuous data and colour, also colour the header row grey."
        n77 = property on="Results Table" class="Tbl (strict)"(error in=w229, "Active Cell"=w228, "Cell BG Color"=u32 16448250, "Value"=w226, "Column Headers[]"=w225) -> (error out=w224:errorcluster)  [unwired: 1 in, 1 out]
        n78 = property on="Results Table" class="Tbl (strict)"(error in=w224, "Active Cell"=w222, "Cell BG Color"=u32 11121611) -> (error out=w223:errorcluster)  [unwired: 1 in, 1 out]
        n79 = call <vilib>:"Add State(s) to Queue__jki_lib_state_machine.vi"("State(s) in (\"\")"=w232) -> ("States Out"=w231:string)  [unwired: 14 in]
      }
      frame "UI: Init Status" {
        w233 = ""  # Status
        w236 = u32 16774001  # Text.Text Colors:BG Color
        w237 = ""  # PassFail
        # "Initialise the status test and passfail text indicator of previous data."
        n80 = property on="PassFail" class="Str"(error in=w238, "Text.BGColor"=w236, "Value"=w237) -> (error out=w234:errorcluster)  [unwired: 1 in, 1 out]
        n81 = property on="Status" class="Str"(error in=w234, "Value"=w233) -> (error out=w235:errorcluster)  [unwired: 1 in, 1 out]
        n82 = call <vilib>:"Add State(s) to Queue__jki_lib_state_machine.vi"("State(s) in (\"\")"=w241) -> ("States Out"=w240:string)  [unwired: 14 in]
      }
      frame "UI: Abort Button" {
        w245 = T7."Disabled and Grayed Out"  # Disabled
        w246 = T7."Enabled"  # Disabled
        # "Enables or disabled the Abort button based on state arguments."
        n83 = Equal?(x=w243, y="Disabled") -> (x = y?=w247:bool)
        n84 = Select(t=w245, s=w247, f=w246) -> (s? t:f=w242:T7)
        n85 = property on="Abort Sequence" class="Bool"(error in=w248, "DisabledEnum"=w242) -> (error out=w249:errorcluster)  [unwired: 1 in, 1 out]
        n86 = call <vilib>:"Add State(s) to Queue__jki_lib_state_machine.vi"("State(s) in (\"\")"=w252) -> ("States Out"=w251:string)  [unwired: 14 in]
      }
      frame "UI: Cursor Set" {
        # "Argument"
        # "Set and Unset Cursor Busy.\n(Usage: \"UI: Cursor Set >> Busy|Idle\")"
        n87 = case shown="\"Busy\"" w253 {
          tunnel: w255 -> [w260 w262]
          tunnel: [w259 w261] -> w254
          frame "Idle", Default {
            n88 = call <vilib>:"Unset Busy.vi"("error in (no error)"=w260) -> ("error out"=w259:errorcluster)  [unwired: 10 in]
          }
          frame "Busy" {
            n89 = call <vilib>:"Set Busy.vi"("error in (no error)"=w262) -> ("error out"=w261:errorcluster)  [unwired: 9 in, 1 out]
          }
        }
        n90 = call <vilib>:"Add State(s) to Queue__jki_lib_state_machine.vi"("State(s) in (\"\")"=w258) -> ("States Out"=w257:string)  [unwired: 14 in]
      }
      frame "UI: Front Panel State" {
        # "Argument"
        # "Set Front Panel Open or Closed\n(Usage: \"UI: Front Panel State >> Open|Close\")"
        n91 = Unbundle By Name(w265) -> ("Core.Current VI Reference"=w264:refnum<vi>)
        n92 = case shown="\"Minimize\", \"Minimized\"" w263 {
          tunnel: w267 -> [w275 w290 w301 w314 w327]
          tunnel: [w277 w291 w303 w316 w329] -> w266
          tunnel: w264 -> [w276 w288 w302 w315 w328]
          frame "Open", "Standard", Default {
            w270 = T1."Standard" ("State")
            n93 = property class="VI"(reference=w276, error in=w275) -> (reference out=w273:refnum<vi>, error out=w274:errorcluster, "FP.State"=w272:T1)
            n94 = Not Equal?(x=w272, y=w270) -> (x != y?=w271:bool)
            n95 = case shown="True" w271 {
              tunnel: [w281 w283] -> w277
              tunnel: w274 -> [w280 w283]
              tunnel: w273 -> [w279 _]
              tunnel: w270 -> [w278 _]
              frame True {
                n96 = invoke class="VI" method="FP.Open"(reference=w279, error in=w280, "Activate"=TRUE, "State"=w278) -> (error out=w281:errorcluster)  [unwired: 1 in, 4 out]
              }
              frame False {
              }
            }
          }
          frame "Close", "Closed" {
            n97 = property class="VI"(reference=w288, error in=w290) -> (reference out=w287:refnum<vi>, error out=w289:errorcluster, "FP.State"=w285:T1)
            n98 = Not Equal?(x=w285, y=T1."Closed" ("Front Panel Window:State")) -> (x != y?=w284:bool)
            n99 = case shown="True" w284 {
              tunnel: [w292 w295] -> w291
              tunnel: w289 -> [w292 w294]
              tunnel: w287 -> [_ w293]
              frame False {
              }
              frame True {
                n100 = invoke class="VI" method="FP.Close"(reference=w293, error in=w294) -> (error out=w295:errorcluster)  [unwired: 1 in, 2 out]
              }
            }
          }
          frame "Hidden", "Hide" {
            w296 = T1."Hidden" ("State")
            n101 = property class="VI"(reference=w302, error in=w301) -> (reference out=w299:refnum<vi>, error out=w300:errorcluster, "FP.State"=w298:T1)
            n102 = Not Equal?(x=w298, y=w296) -> (x != y?=w297:bool)
            n103 = case shown="True" w297 {
              tunnel: [w307 w308] -> w303
              tunnel: w300 -> [w306 w308]
              tunnel: w299 -> [w305 _]
              tunnel: w296 -> [w304 _]
              frame True {
                n104 = invoke class="VI" method="FP.Open"(reference=w305, error in=w306, "State"=w304) -> (error out=w307:errorcluster)  [unwired: 2 in, 4 out]
              }
              frame False {
              }
            }
          }
          frame "Minimize", "Minimized" {
            w309 = T1."Minimized" ("State")
            n105 = property class="VI"(reference=w315, error in=w314) -> (reference out=w312:refnum<vi>, error out=w313:errorcluster, "FP.State"=w311:T1)
            n106 = Not Equal?(x=w311, y=w309) -> (x != y?=w310:bool)
            n107 = case shown="True" w310 {
              tunnel: [w320 w321] -> w316
              tunnel: w313 -> [w319 w321]
              tunnel: w312 -> [w318 _]
              tunnel: w309 -> [w317 _]
              frame True {
                n108 = invoke class="VI" method="FP.Open"(reference=w318, error in=w319, "State"=w317) -> (error out=w320:errorcluster)  [unwired: 2 in, 4 out]
              }
              frame False {
              }
            }
          }
          frame "Maximize", "Maximized" {
            w322 = T1."Maximized" ("State")
            n109 = property class="VI"(reference=w328, error in=w327) -> (reference out=w325:refnum<vi>, error out=w326:errorcluster, "FP.State"=w324:T1)
            n110 = Not Equal?(x=w324, y=w322) -> (x != y?=w323:bool)
            n111 = case shown="True" w323 {
              tunnel: [w333 w334] -> w329
              tunnel: w326 -> [w332 w334]
              tunnel: w325 -> [w331 _]
              tunnel: w322 -> [w330 _]
              frame True {
                n112 = invoke class="VI" method="FP.Open"(reference=w331, error in=w332, "State"=w330) -> (error out=w333:errorcluster)  [unwired: 2 in, 4 out]
              }
              frame False {
              }
            }
          }
        }
        n113 = call <vilib>:"Add State(s) to Queue__jki_lib_state_machine.vi"("State(s) in (\"\")"=w269) -> ("States Out"=w268:string)  [unwired: 14 in]
      }
      frame "---------- Macro ----------" {
        # "Do not put any code in this frame.\n(It is a separator no-op. You can make a copy of this frame to create a new Macro frame)"
        n114 = call <vilib>:"Add State(s) to Queue__jki_lib_state_machine.vi"("State(s) in (\"\")"=w338) -> ("States Out"=w337:string)  [unwired: 14 in]
      }
      frame "Macro: Initialize" {
        w339 = "Data: Initialize\nInitialize Core Data\nUI: Initialize\nUI: Init Results Table\nUI: Init Status\nUI: Run Button >> Disabled\nUI: Abort Button >> Disabled\nUI: Front Panel State >> Open"  # Data: Initialize Initialize Core Data UI: Initialize UI: Init Results Table UI: Init Status UI: Run Button >> Disabled UI: Abort Button >> Disabled UI: Front Panel State >> Open
        # "Initialization Macro\n(This is called once, when the VI starts)"
        n115 = call <vilib>:"Add State(s) to Queue__jki_lib_state_machine.vi"("State(s) in Front (\"\")"=w339, "State(s) in (\"\")"=w343) -> ("States Out"=w342:string)  [unwired: 13 in]
      }
      frame "Macro: Load Sequence" {
        # "Macro to load the sequence file."
        n116 = call <vilib>:"Add State(s) to Queue__jki_lib_state_machine.vi"("State(s) in Front (\"\")"="Sequence: Load File\nSequence: Get Sequence Name\nSequence: Check Sequence\nSequence: Test Path Array\nSequence: Set Limits Path", "State(s) in (\"\")"=w348) -> ("States Out"=w347:string)  [unwired: 13 in]
      }
      frame "Macro: Run Sequence" {
        # "Macro to run a sequence, this also calls the run test macro to execute each test."
        n117 = call <vilib>:"Add State(s) to Queue__jki_lib_state_machine.vi"("State(s) in Front (\"\")"="Results Log: Scan Barcode\nUI: Abort Button>>Enable\nResults Log: Start Sequence Time\nResults Log: Set Results Path\nResults Log: Build Results Header\nUI: Init Results Table\nUI: Init Status\nUI: Tab Control>>Results\nMacro: Run Test", "State(s) in (\"\")"=w353) -> ("States Out"=w352:string)  [unwired: 13 in]
      }
      frame "Macro: End Sequence" {
        # "Macro to run after each test sequence is executed."
        n118 = call <vilib>:"Add State(s) to Queue__jki_lib_state_machine.vi"("State(s) in Front (\"\")"="Testing: Close References\nUI: Tab Control>>Sequence\nResults Log: End Sequence Time\nUI: Update Status\nResults Log: Rename Results File\nSequence: Reset Sequence Data\nUI: Abort Button>>Disabled", "State(s) in (\"\")"=w358) -> ("States Out"=w357:string)  [unwired: 13 in]
      }
      frame "Macro: Abort Sequence" {
        # "Macro to run if abort button is pressed."
        n119 = call <vilib>:"Add State(s) to Queue__jki_lib_state_machine.vi"("State(s) in Front (\"\")"="Testing: Close References\nUI: Tab Control>>Sequence\nResults Log: End Sequence Time\nResults Log: Rename Results File\nSequence: Reset Sequence Data\nUI: Abort Button>>Disabled\nSequence: Abort Sequence", "State(s) in (\"\")"=w363) -> ("States Out"=w362:string)  [unwired: 13 in]
      }
      frame "Macro: Run Test" {
        # "Macro to loop for each test to execute in the test sequence. Call idle to see if abort button has been pressed."
        n120 = call <vilib>:"Add State(s) to Queue__jki_lib_state_machine.vi"("State(s) in Front (\"\")"="Testing: Test Timer Start\nTesting: Call Test\nTesting: Test Timer Stop\nResults Log: Add Test Time\nResults Log: Update Results Display\nTesting: Check Stop On Fail\nIdle\nTesting: Check Sequence End", "State(s) in (\"\")"=w368) -> ("States Out"=w367:string)  [unwired: 13 in]
      }
      frame "Macro: Exit" {
        # "Exit Macro\n(This is called once, when the VI exits)"
        n121 = Unbundle By Name(w375) -> ("Core.Close Panel on Exit?"=w370:bool)
        n122 = call <vilib>:"Conditional State String__jki_lib_state_machine.vi"("Do State(s)?"=w370, "State"="UI: Front Panel State >> Close") -> ("State Out"=w369:string)  [unwired: 7 in]
        n123 = call <vilib>:"Add State(s) to Queue__jki_lib_state_machine.vi"("State(s) in (\"\")"=w369, "State(s) at Back (\"\")"="UI: Uninitialize\nData: Cleanup\nExit") -> ("States Out"=w373:string)  [unwired: 13 in]
        n124 = call <vilib>:"Add State(s) to Queue__jki_lib_state_machine.vi"("State(s) in Front (\"\")"=w373, "State(s) in (\"\")"=w377) -> ("States Out"=w376:string)  [unwired: 13 in]
      }
      frame "---------- Sequence ----------" {
        # "Template Separator\n(You can make a copy of, or modify, this frame)"
        n125 = call <vilib>:"Add State(s) to Queue__jki_lib_state_machine.vi"("State(s) in (\"\")"=w381) -> ("States Out"=w380:string)  [unwired: 14 in]
      }
      frame "Sequence: Load File" {
        # "Needs to handle if the load sequence is cancelled\n, doesn't currently."
        # "Prompts the user to select the sequence file to run. Also formats the array into something to display on the FP."
        n126 = call <userlib>:"Current VIs Parent Directory__ogtk.vi"() -> ("Parent Directory (+ Relative)"=w386:path)  [unwired: 5 in]
        n127 = Build Path(base path=w386, name or relative path="Sequence") -> (appended path=w388:path)
        n128 = call "File Dialog"("start path"=w388, "prompt"="Load Sequence File", "error in"=w392, "pattern (all files)"="*.csv", "pattern label"="Sequence File") -> ("selected path"=w389:path, "error out"=w393:errorcluster)  [unwired: 7 in, 2 out]
        n129 = case shown="No Error" w393 {
          selector: w393 -> [w403 w405]
          tunnel: w389 -> [w402 _]
          tunnel: [w401 w405] -> w384
          tunnel: [w400 string[] []] -> w383
          frame No Error {
            w399 = ","  # delimiter (\t)
            n130 = call-poly <vilib>:"Read Delimited Spreadsheet.vi"("file path (dialog if empty)"=w402, "error in (no error)"=w403, "delimiter (\\t)"=w399) -> ("first row"=w400:string[], "error out"=w401:errorcluster)  [unwired: 7 in, 4 out]
          }
          frame Error {
          }
        }
        n131 = Bundle By Name(cluster=w391, "File Paths.Seq File Path"=w389, "Sequence Array"=w383) -> (w390:T3)
        n132 = call "Sequence Array Formatting.vi"("Sequence Array"=w383, "error in"=w384) -> ("Formatted Sequence"=→"Sequence":string, "error out"=w385:errorcluster)  [unwired: 12 in]
        n133 = call <vilib>:"Add State(s) to Queue__jki_lib_state_machine.vi"("State(s) in (\"\")"=w398) -> ("States Out"=w397:string)  [unwired: 14 in]
      }
      frame "Sequence: Check Sequence" {
        # "This is legacy, not sure if this is needed now\nNeeds review"
        # "Check if the sequence is valid and enables the run button if it is."
        n134 = Unbundle By Name(w408) -> ("Sequence Name"=w407:string)
        n135 = Equal?(x=w407, y="") -> (x = y?=w410:bool)
        n136 = case shown="True" w410 {
          tunnel: ["UI: Run Button>>Enable\n#UI: Abort Button>>Enable" "UI: Run Button>>Disabled\nUI: Abort Button>>Disabled"] -> w406
          frame False {
          }
          frame True {
            n137 = One Button Dialog(message="ERROR: Sequence name is set to \"None\".") -> ()  [unwired: 1 in, 1 out]
          }
        }
        n138 = call <vilib>:"Add State(s) to Queue__jki_lib_state_machine.vi"("State(s) in (\"\")"=w413, "State(s) at Back (\"\")"=w406) -> ("States Out"=w412:string)  [unwired: 13 in]
      }
      frame "Sequence: Get Sequence Name" {
        # "Strips the sequence name based on the sequence file path."
        n139 = Unbundle By Name(w422) -> ("File Paths.Seq File Path"=w419:path)
        n140 = Strip Path(path=w419) -> (name=w418:string)  [unwired: 1 out]
        n141 = call-poly <userlib>:"Strip Path Extension__ogtk.vi"("path"=w418) -> ("root"=w417:string)  [unwired: 1 out]
        "Sequence Name" <- w417
        n142 = Bundle By Name(cluster=w422, "Sequence Name"=w417) -> (w421:T3)
        n143 = call <vilib>:"Add State(s) to Queue__jki_lib_state_machine.vi"("State(s) in (\"\")"=w424) -> ("States Out"=w423:string)  [unwired: 14 in]
      }
      frame "Sequence: Abort Sequence" {
        # "Aborts the sequence, clear the state queue"
        n144 = property on="PassFail" class="Str"(error in=w429, "Text.BGColor"=u32 16767232 ("Text.Text Colors:BG Color"), "Value"="Aborted" ("PassFail")) -> (error out=w426:errorcluster)  [unwired: 1 in, 1 out]
        n145 = call <vilib>:"Add State(s) to Queue__jki_lib_state_machine.vi"() -> ("States Out"=w430:string)  [unwired: 15 in]
      }
      frame "Sequence: Reset Sequence Data" {
        # "Resets the sequence data"
        n146 = Bundle By Name(cluster=w437, "Test Index"=0, "Fail"=FALSE, "Abort"=FALSE) -> (w436:T3)
        n147 = call <vilib>:"Add State(s) to Queue__jki_lib_state_machine.vi"("State(s) in (\"\")"=w431) -> ("States Out"=w438:string)  [unwired: 14 in]
      }
      frame "Sequence: Set Limits Path" {
        # "Sets the sequence limits file path based on the sequence file name (as they are intrinsically linked)."
        n148 = Unbundle By Name(w452) -> ("File Paths.Seq File Path"=w449:path)
        n149 = Strip Path(path=w449) -> (stripped path=w445:path, name=w448:string)
        n150 = Strip Path(path=w445) -> (stripped path=w444:path)  [unwired: 1 out]
        n151 = call-poly <userlib>:"Strip Path Extension__ogtk.vi"("path"=w448) -> ("root"=w439:string)  [unwired: 1 out]
        n152 = call <vilib>:"Space Constant.vi"() -> ("String"=w447:string)
        n153 = Concatenate Strings(w439, w447, "Limits.csv") -> (w441:string)
        n154 = Build Path(base path=w444, name or relative path="Limits") -> (appended path=w442:path)
        n155 = Build Path(base path=w442, name or relative path=w441) -> (appended path=w440:path)
        n156 = Bundle By Name(cluster=w452, "File Paths.Limits File Path"=w440) -> (w451:T3)
        n157 = call <vilib>:"Add State(s) to Queue__jki_lib_state_machine.vi"("State(s) in (\"\")"=w454) -> ("States Out"=w453:string)  [unwired: 14 in]
      }
      frame "Sequence: Test Path Array" {
        # "Builds an array of file paths based on the sequence array."
        n158 = Unbundle By Name(w460) -> ("Sequence Array"=w457:string[])
        n159 = for {
          tunnel: w458 -> [w464]
          tunnel: w457 -> [w469] mode=indexing
          tunnel: [w465] -> w456 mode=indexing
          tunnel: [w464] -> w455
          n160 = call <userlib>:"Current VIs Parent Directory__ogtk.vi"() -> ("Parent Directory (+ Relative)"=w463:path)  [unwired: 5 in]
          n161 = Concatenate Strings(w469, ".vi") -> (w466:string)
          n162 = Build Path(base path=w463, name or relative path="Tests") -> (appended path=w467:path)
          n163 = Build Path(base path=w467, name or relative path=w466) -> (appended path=w465:path)
        }
        n164 = Bundle By Name(cluster=w460, "File Paths.Test File Path Array"=w456) -> (w459:T3)
        n165 = call <vilib>:"Add State(s) to Queue__jki_lib_state_machine.vi"("State(s) in (\"\")"=w462) -> ("States Out"=w461:string)  [unwired: 14 in]
      }
      frame "---------- Results Log ----------" {
        # "Template Separator\n(You can make a copy of, or modify, this frame)"
        n166 = call <vilib>:"Add State(s) to Queue__jki_lib_state_machine.vi"("State(s) in (\"\")"=w474) -> ("States Out"=w473:string)  [unwired: 14 in]
      }
      frame "Results Log: Set Results Path" {
        w475 = TRUE  # replace all? (F)
        w480 = "-"
        # "Set constant for now, can be configurable later"
        # "Build a file path for the results based upon the serial number, test time and date."
        n167 = Unbundle By Name(w487) -> ("Serial Number"=w486:string, "Start Seq TimeStamp.Start Seq Time"=w482:string, "Start Seq TimeStamp.Start Seq Date"=w478:string)
        n168 = Search and Replace String(replace all?=w475, input string=w482, search string=":") -> (result string=w481:string)  [unwired: 5 in, 3 out]
        n169 = Search and Replace String(replace all?=w475, input string=w478, search string="/") -> (result string=w477:string)  [unwired: 5 in, 3 out]
        n170 = Concatenate Strings(w486, w480, w481, w480, w477, ".csv") -> (w484:string)
        n171 = Build Path(base path=path "C:/results", name or relative path=w484) -> (appended path=w483:path)
        n172 = Bundle By Name(cluster=w487, "File Paths.Results File Path"=w483) -> (w490:T3)
        n173 = call <vilib>:"Add State(s) to Queue__jki_lib_state_machine.vi"("State(s) in (\"\")"=w492) -> ("States Out"=w491:string)  [unwired: 14 in]
      }
      frame "Results Log: Rename Results File" {
        # "Change the results file name to include the final test status."
        n174 = Unbundle By Name(w511) -> ("File Paths.Results File Path"=w509:path, "Abort"=w496:bool, "Fail"=w497:bool)
        n175 = Strip Path(path=w509) -> (stripped path=w502:path, name=w507:string)
        n176 = call-poly <userlib>:"Strip Path Extension__ogtk.vi"("path"=w507) -> ("root"=w504:string, "extension"=w503:string)
        n177 = Select(t="-Fail", s=w497, f="-Pass") -> (s? t:f=w495:string)
        n178 = Select(t="-Aborted", s=w496, f=w495) -> (s? t:f=w494:string)
        n179 = Concatenate Strings(w504, w494, ".", w503) -> (w501:string)
        n180 = Build Path(base path=w502, name or relative path=w501) -> (appended path=w500:path)
        n181 = call-poly <userlib>:"FILE Rename__ogtk.vi"("error in (no error)"=w510, "overwrite (F)"=TRUE, "source path"=w509, "target path"=w500) -> ("error out"=w499:errorcluster)  [unwired: 6 in, 1 out]
        n182 = call <vilib>:"Add State(s) to Queue__jki_lib_state_machine.vi"("State(s) in (\"\")"=w513) -> ("States Out"=w512:string)  [unwired: 14 in]
      }
      frame "Results Log: Start Sequence Time" {
        w515 = "%d/%m/%y"  # time format string (%c)
        w519 = "%H:%M:%S"  # time format string (%c)
        # "Captures the date and time for the start of the test."
        n183 = Format Date/Time String(time format string (%c)=w515) -> (date/time string=w514:string)  [unwired: 2 in]
        n184 = Format Date/Time String(time format string (%c)=w519) -> (date/time string=w516:string)  [unwired: 2 in]
        n185 = Bundle By Name(cluster=w518, "Start Seq TimeStamp.Start Seq Time"=w516, "Start Seq TimeStamp.Start Seq Date"=w514) -> (w517:T3)
        n186 = call <vilib>:"Add State(s) to Queue__jki_lib_state_machine.vi"("State(s) in (\"\")"=w522) -> ("States Out"=w521:string)  [unwired: 14 in]
      }
      frame "Results Log: Update Results Display" {
        w525 = "Fail"  # element
        w529 = 7  # index
        w535 = 8  # index
        w537 = ","  # delimiter (\t)
        # "Strip out the test details \nstuff at the begining of \nresults file"
        # "Update the results display from the results log, colours in the status coloum with the appropriate colour."
        n187 = Unbundle By Name(w528) -> ("File Paths.Results File Path"=w533:path)
        n188 = call-poly <vilib>:"Read Delimited Spreadsheet.vi"("file path (dialog if empty)"=w533, "error in (no error)"=w534, "delimiter (\\t)"=w537) -> ("all rows"=w536:string[][], "error out"=w530:errorcluster)  [unwired: 7 in, 4 out]
        n189 = Array Subset(array=w536, index (row)=w535) -> (w532:string[][])  [unwired: 3 in]
        "Results Table" <- w532
        n190 = Index Array(array=w532, index (col)=w529) -> (element=w526:string[])  [unwired: 1 in]
        n191 = for {
          tunnel: [w544] -> w531
          tunnel: w526 -> [w547] mode=indexing
          tunnel: w530 -> [w543]
          i -> [w546]
          w545 = 7  # Column
          n192 = Equal?(x=w547, y="Pass") -> (x = y?=w540:bool)
          n193 = Select(t=u32 51250, s=w540, f=u32 15663143) -> (s? t:f=w542:u32)
          n194 = Bundle(w546, "Column"=w545) -> (w541:cluster{i32, "Column":i32})  [unwired: 1 in]
          n195 = property on="Results Table" class="Tbl (strict)"(error in=w543, "Active Cell"=w541, "Cell BG Color"=w542) -> (error out=w544:errorcluster)  [unwired: 1 in, 1 out]
        }
        n196 = Search 1D Array(1D array=w526, element=w525) -> (index of element=w524:i32)  [unwired: 1 in]
        n197 = Greater Or Equal To 0?(x=w524) -> (x >= 0?=w523:bool)
        n198 = Bundle By Name(cluster=w528, "Fail"=w523) -> (w527:T3)
        n199 = call <vilib>:"Add State(s) to Queue__jki_lib_state_machine.vi"("State(s) in (\"\")"=w539) -> ("States Out"=w538:string)  [unwired: 14 in]
      }
      frame "Results Log: Add Test Time" {
        w567 = "s"  # string
        w568 = ","  # string
        w575 = TRUE  # multiline? (F)
        w557 = "(.*)$"  # search string
        # "Replace the line to include the\ntest time"
        # "Searching for the first instance\nof test name, will return the\nwhole line"
        # "Formatting the test time"
        # "Adds the test time to the results log. Horrendous."
        n200 = Unbundle By Name(w578) -> ("Test Time"=w570:dbl, "Sequence Array"=w556:string[], "Test Index"=w555:i32, "File Paths.Results File Path"=w559:path)
        n201 = Decrement(x=w555) -> (x-1=w554:i32)
        n202 = Open/Create/Replace File(file path (use dialog)=w559, error in=w571) -> (refnum out=w577:refnum<file>, error out=w576:errorcluster)  [unwired: 4 in, 1 out]
        n203 = Index Array(array=w556, index=w554) -> (element=w553:string)
        n204 = Read from Text File(file (use dialog)=w577, error in=w576) -> (refnum out=w560:refnum<file>, text=w574:string, error out=w561:errorcluster)  [unwired: 2 in, 1 out]
        n205 = Number To Fractional String(number=w570) -> (F-format string=w569:string)  [unwired: 3 in]
        n206 = Concatenate Strings(w553, w557) -> (w558:string)
        n207 = xnode "Match Regular Expression"("input string"=w574, "regular expression"=w558, "multiline? (F)"=w575) -> ("whole match"=w573:string, "offset past match"=w552:i32)  [unwired: 3 in, 3 out]
        n208 = Concatenate Strings(w568, w569, w567) -> (w566:string)
        n209 = Greater Or Equal To 0?(x=w552) -> (x >= 0?=w551:bool)
        n210 = Concatenate Strings(w573, w566) -> (w572:string)
        n211 = Search and Replace String(input string=w574, search string=w573, replace string=w572) -> (result string=w565:string)  [unwired: 5 in, 3 out]
        n212 = case shown="True" w551 {
          tunnel: w565 -> [_ w590]
          tunnel: [w581 w589] -> w564
          tunnel: [w582 w588] -> w563
          tunnel: w561 -> [w581 w586]
          tunnel: w560 -> [w582 w585]
          frame False {
            # "Can't find the test name\nin the results so do nothing"
          }
          frame True {
            w583 = i64 0  # size (in bytes)
            # "Overwrite whole file"
            n213 = Set File Size(4:w586, 6:w583, 7:w585) -> (0:w587:errorcluster, 3:w584:refnum<file>)
            n214 = Write to Text File(file (use dialog)=w584, text=w590, error in=w587) -> (refnum out=w588:refnum<file>, error out=w589:errorcluster)  [unwired: 1 in, 1 out]
          }
        }
        n215 = Close File(refnum=w563, error in=w564) -> (error out=w562:errorcluster)  [unwired: 1 out]
        n216 = call <vilib>:"Add State(s) to Queue__jki_lib_state_machine.vi"("State(s) in (\"\")"=w580) -> ("States Out"=w579:string)  [unwired: 14 in]
      }
      frame "Results Log: End Sequence Time" {
        w711 = "%H:%M:%S"  # time format string (%c)
        # "Captures the date and time for the start of the test."
        n217 = Format Date/Time String(time format string (%c)=w711) -> (date/time string=w708:string)  [unwired: 2 in]
        n218 = Bundle By Name(cluster=w710, "End Seq Time"=w708) -> (w709:T3)
        n219 = call <vilib>:"Add State(s) to Queue__jki_lib_state_machine.vi"("State(s) in (\"\")"=w714) -> ("States Out"=w713:string)  [unwired: 14 in]
      }
      frame "Results Log: Build Results Header" {
        w718 = TRUE  # transpose? (no:F)
        w719 = FALSE  # append to file? (new file:F)
        # "Builds a header for the results log file."
        n220 = Unbundle By Name(w728) -> ("File Paths.Results File Path"=w715:path, "Operator"=w726:string, "Serial Number"=w725:string, "Start Seq TimeStamp.Start Seq Date"=w717:string, "Start Seq TimeStamp.Start Seq Time"=w716:string, "Sequence Name"=w724:string)
        n221 = call "Build Text"("Time"=w716, "Operator"=w726, "Serial Number"=w725, "Date"=w717, "error in (no error)"=w727, "Sequence Name"=w724) -> ("Result"=w723:string, "error out"=w721:errorcluster)  [unwired: 8 in]
        n222 = call <userlib>:"Multi-line String to Array__ogtk.vi"("string"=w723) -> ("lines"=w720:string[])
        n223 = Bundle By Name(cluster=w728, "Status"=w723) -> (w729:T3)
        n224 = call-poly <vilib>:"Write Delimited Spreadsheet.vi"("file path (dialog if empty)"=w715, "1D data"=w720, "append to file? (new file:F)"=w719, "error in (no error)"=w721, "transpose? (no:F)"=w718) -> ("error out"=w722:errorcluster)  [unwired: 9 in, 1 out]
        n225 = call <vilib>:"Add State(s) to Queue__jki_lib_state_machine.vi"("State(s) in (\"\")"=w731) -> ("States Out"=w730:string)  [unwired: 14 in]
      }
      frame "Results Log: Scan Barcode" {
        # "Prompts the user to input thier name and scan serial barcode for traceability. Operator name persists so it is not required to be input every time."
        n226 = Unbundle By Name(w744) -> ("Operator"=w741:string)
        n227 = call "Scan Barcode.vi"("Operator"=w741, "error in"=w742) -> ("Operator Name Out"=w736:string, "Serial Number Out"=w735:string, "Cancelled?"=w740:bool, "error out"=w739:errorcluster)  [unwired: 10 in]
        n228 = case shown="False" w740 {
          tunnel: w739 -> [w746 w751]
          tunnel: [w746 w751] -> w738
          tunnel: w737 -> [w747 _]
          tunnel: w736 -> [w748 _]
          tunnel: w735 -> [w749 _]
          tunnel: [w749 w750] -> w734
          tunnel: [w748 w750] -> w733
          tunnel: [w747 w750] -> w732
          frame False {
          }
          frame True {
            w750 = "" ("Remaining States")
          }
        }
        "Serial Number" <- w734
        "Operator" <- w733
        n229 = Bundle By Name(cluster=w744, "Operator"=w733, "Serial Number"=w734) -> (w743:T3)
        n230 = call <vilib>:"Add State(s) to Queue__jki_lib_state_machine.vi"("State(s) in (\"\")"=w732) -> ("States Out"=w745:string)  [unwired: 14 in]
      }
      frame "---------- Testing ----------" {
        # "Template Separator\n(You can make a copy of, or modify, this frame)"
        n231 = call <vilib>:"Add State(s) to Queue__jki_lib_state_machine.vi"("State(s) in (\"\")"=w755) -> ("States Out"=w754:string)  [unwired: 14 in]
      }
      frame "Testing: Check Sequence End" {
        # "Check to see if all tests in teh sequence array have been executed, repeat loop if not, other wise run end sequence macro."
        n232 = Unbundle By Name(w765) -> ("Abort"=w757:bool, "Test Index"=w763:i32, "Sequence Array"=w764:string[])
        n233 = Array Size(array=w764) -> (size(s)=w762:i32)
        n234 = Equal?(x=w763, y=w762) -> (x = y?=w758:bool)
        n235 = Or(x=w757, y=w758) -> (x .or. y?=w756:bool)
        n236 = call-poly <vilib>:"Select State(s)__jki_lib_state_machine.vi"("State(s) if True (\"\")"="Macro: End Sequence", "Select"=w756, "State(s) if False (\"\")"="Macro: Run Test") -> ("States Out"=w759:string)  [unwired: 12 in]
        n237 = call <vilib>:"Add State(s) to Queue__jki_lib_state_machine.vi"("State(s) in (\"\")"=w768, "State(s) at Back (\"\")"=w759) -> ("States Out"=w767:string)  [unwired: 13 in]
      }
      frame "Testing: Check Stop On Fail" {
        # "If stop on fail is enabled and the last test failed, run the last step in the sequence which should be shutdown/cleanup."
        n238 = Unbundle By Name(w776) -> ("Sequence Array"=w777:string[], "Fail"=w779:bool, "SOF"=w778:bool, "Test Index"=w772:i32)
        n239 = And(x=w779, y=w778) -> (x .and. y?=w773:bool)
        n240 = Array Size(array=w777) -> (size(s)=w780:i32)
        n241 = Decrement(x=w780) -> (x-1=w771:i32)
        n242 = Less?(x=w772, y=w771) -> (x < y?=w769:bool)
        n243 = And(x=w773, y=w769) -> (x .and. y?=w770:bool)
        n244 = Select(t=w771, s=w770, f=w772) -> (s? t:f=w774:i32)
        n245 = Bundle By Name(cluster=w776, "Test Index"=w774) -> (w775:T3)
        n246 = call <vilib>:"Add State(s) to Queue__jki_lib_state_machine.vi"("State(s) in (\"\")"=w783) -> ("States Out"=w782:string)  [unwired: 14 in]
      }
      frame "Testing: Test Timer Start" {
        # "Naughtily have used the same variable\nfor start time and total time of test."
        # "Capture the time for the begining of each test."
        n247 = Get Date/Time In Seconds() -> (seconds since 1Jan1904=w787:timestamp)
        n248 = To Double Precision Float(number=w787) -> (double precision float=w784:dbl)
        n249 = Bundle By Name(cluster=w786, "Test Time"=w784) -> (w785:T3)
        n250 = call <vilib>:"Add State(s) to Queue__jki_lib_state_machine.vi"("State(s) in (\"\")"=w790) -> ("States Out"=w789:string)  [unwired: 14 in]
      }
      frame "Testing: Test Timer Stop" {
        # "Naughtily have used the same variable\nfor start time and total time of test."
        # "Capture the time for the end of each test. Calculate the timein seconds."
        n251 = Unbundle By Name(w793) -> ("Test Time"=w794:dbl)
        n252 = Get Date/Time In Seconds() -> (seconds since 1Jan1904=w796:timestamp)
        n253 = To Double Precision Float(number=w796) -> (double precision float=w795:dbl)
        n254 = Subtract(x=w795, y=w794) -> (x-y=w791:dbl)
        n255 = Bundle By Name(cluster=w793, "Test Time"=w791) -> (w792:T3)
        n256 = call <vilib>:"Add State(s) to Queue__jki_lib_state_machine.vi"("State(s) in (\"\")"=w799) -> ("States Out"=w798:string)  [unwired: 14 in]
      }
      frame "Testing: Call Test" {
        # "Collect references rather than\nclose them. Keeps any FGV data \nin memory."
        # "Call each test by reference using the test file path. Unfortunately this means that each test will need to be strictly type def (each test vi must have the same pattern and inputs and outputs). Increase the index so that the next test will be in the next loop."
        n257 = Unbundle By Name(w807) -> ("Reference Array"=w802:refnum<vi>[], "File Paths.Limits File Path"=w811:path, "File Paths.Results File Path"=w810:path, "File Paths.Test File Path Array"=w809:path[], "Test Index"=w804:i32)
        n258 = Index Array(array=w809, index=w804) -> (element=w808:path)
        n259 = Open VI Reference(type specifier VI Refnum (for type only)=refnum<vi> refnum, vi path=w808, error in (no error)=w812) -> (vi reference=w815:refnum<vi>, error out=w814:errorcluster)  [unwired: 3 in]
        n260 = Increment(x=w804) -> (x+1=w805:i32)
        n261 = call-by-ref "?"(reference=w815, "Limits File Path"=w811, "Results File Path"=w810, "error in"=w814) -> (reference out=w801:refnum<vi>, "error out"=w813:errorcluster)  [unwired: 13 in, 1 out]
        n262 = Build Array (concatenate)(w802, w801) -> (w800:refnum<vi>[])
        n263 = Bundle By Name(cluster=w807, "Test Index"=w805, "Reference Array"=w800) -> (w806:T3)
        n264 = call <vilib>:"Add State(s) to Queue__jki_lib_state_machine.vi"("State(s) in (\"\")"=w817) -> ("States Out"=w816:string)  [unwired: 14 in]
      }
      frame "Testing: Close References" {
        # "Close test VI references opened during the sequence run."
        n265 = Unbundle By Name(w823) -> ("Reference Array"=w818:refnum<vi>[])
        n266 = for {
          tunnel: [w828] -> w820
          tunnel: w819 -> [w827]
          tunnel: w818 -> [w826] mode=indexing
          n267 = Close Reference(reference=w826, error in (no error)=w827) -> (error out=w828:errorcluster)
        }
        n268 = Bundle By Name(cluster=w823, "Reference Array"=refnum<vi>[] []) -> (w822:T3)
        n269 = call <vilib>:"Add State(s) to Queue__jki_lib_state_machine.vi"("State(s) in (\"\")"=w825) -> ("States Out"=w824:string)  [unwired: 14 in]
      }
    }
  }
